vi "Tab Key Process.vi"(4 "CurPage Ctrl #n":refnum<vi>, 5 "Char":i16, 6 "CurPage Ctrl #1":refnum<vi>, 7 "Shift":bool, 9 "Help":refnum<vi>, 10 "Next":refnum<vi>, 11 "Back":refnum<vi>) -> (3 "Discard Key Down Event?":bool)   [LabVIEW 2021]
uses:
  <vilib>/Utility/traverseref.llb/TRef TravTarget.ctl
  <vilib>/Utility/traverseref.llb/VI Scripting - Traverse.lvlib
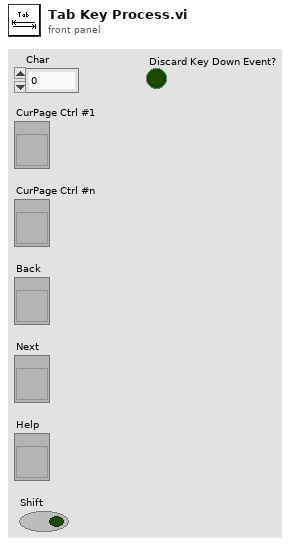
[diagram p1: front panel]
types:
  T1 = typedef "TRef TravTarget.ctl" = enum16{"FP", "BD", "Other"}
  T2 = enum8{"Enabled", "Disabled", "Disabled and Grayed Out"}
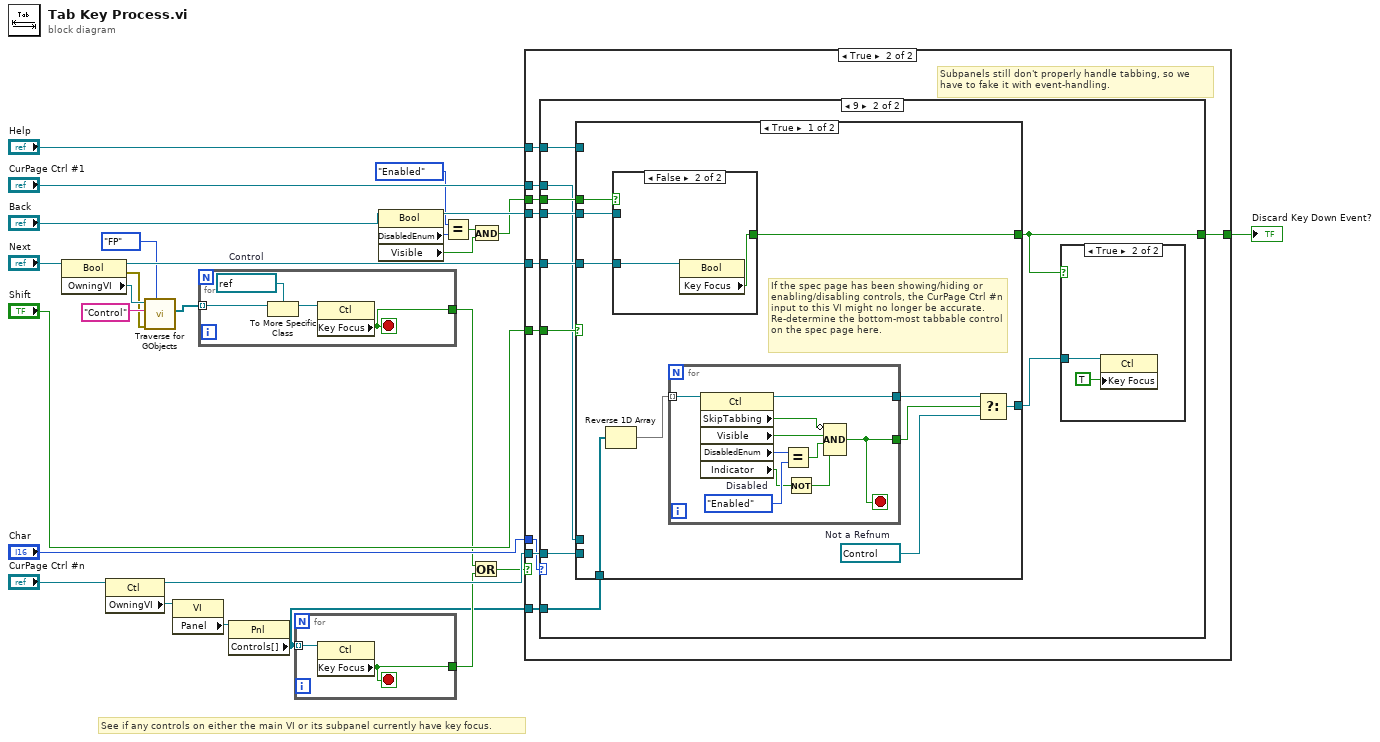
[diagram p0: block diagram]
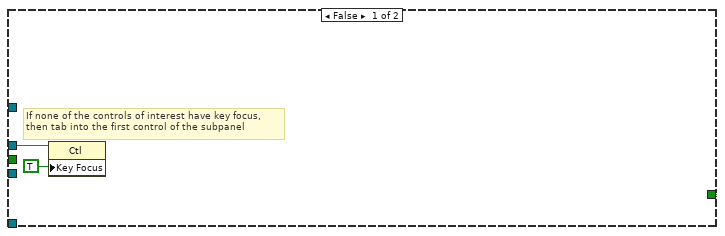
[diagram p2: hidden frame]
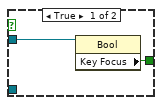
[diagram p5: hidden frame]
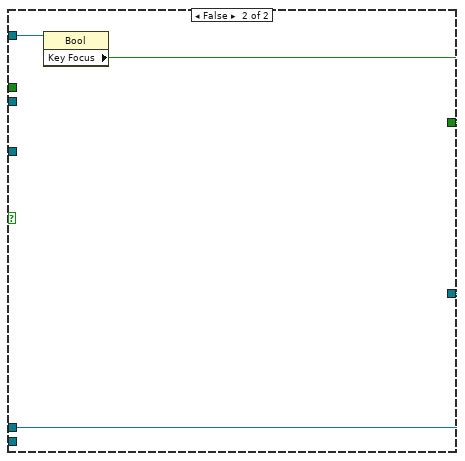
[diagram p6: hidden frame]
diagram:
  # "See if any controls on either the main VI or its subpanel currently have key focus."
  n1 = property class="Bool"(reference="Next") -> (reference out=w13:refnum<vi>, error out=w3:errorcluster, "OwningVI"=w6:refnum<vi>)  [unwired: 1 in]
  n2 = property class="Ctl"(reference="CurPage Ctrl #n") -> (reference out=w12:refnum<vi>, "OwningVI"=w10:refnum<vi>)  [unwired: 1 in, 1 out]
  n3 = call <vilib>:"Traverse for GObjects.vi"("Traverse Target"=TRef_TravTarget."FP", "error in (no error)"=w3, "Class Name"="Control", "VI Refnum"=w6) -> ("References"=w2:refnum<vi>[])  [unwired: 4 in, 3 out]
  n4 = property class="VI"(reference=w10) -> ("Panel"=w11:refnum<vi>)  [unwired: 1 in, 2 out]
  n5 = for {
    tunnel: w2 -> [w29] mode=indexing
    tunnel: [w31] -> w8
    stop <- w31 stop-if-true
    w30 = refnum<vi> refnum  # Control
    n6 = To More Specific Class(target class=w30, reference=w29) -> (specific class reference=w28:refnum<vi>)  [unwired: 1 in, 1 out]
    n7 = property class="Ctl"(reference=w28) -> ("Key Focus"=w31:bool)  [unwired: 1 in, 2 out]
  }
  n8 = property class="Pnl"(reference=w11) -> ("Controls[]"=w1:refnum<vi>[])  [unwired: 1 in, 2 out]
  n9 = for {
    tunnel: w1 -> [w33] mode=indexing
    tunnel: [w32] -> w9
    stop <- w32 stop-if-true
    n10 = property class="Ctl"(reference=w33) -> ("Key Focus"=w32:bool)  [unwired: 1 in, 2 out]
  }
  n11 = property on="Property Node" class="Bool"(reference="Back") -> (reference out=w23:refnum<vi>, "DisabledEnum"=w17:T2, "Visible"=w20:bool)  [unwired: 1 in, 1 out]
  n12 = Equal?(x=T2."Enabled", y=w17) -> (x = y?=w19:bool)
  n13 = Or(x=w8, y=w9) -> (x .or. y?=w7:bool)
  n14 = And(x=w19, y=w20) -> (x .and. y?=w21:bool)
  n15 = case shown="True" w7 {
    tunnel: "CurPage Ctrl #1" -> [w36 w46]
    tunnel: w12 -> [_ w45]
    tunnel: "Help" -> [_ w44]
    tunnel: w13 -> [_ w43]
    tunnel: w23 -> [_ w42]
    tunnel: w21 -> [_ w41]
    tunnel: [TRUE ("Key Focus") w40] -> w16
    tunnel: "Shift" -> [_ w39]
    tunnel: "Char" -> [_ w38]
    tunnel: w1 -> [_ w37]
    frame False {
      # "If none of the controls of interest have key focus,\nthen tab into the first control of the subpanel"
      n16 = property class="Ctl"(reference=w36, "Key Focus"=TRUE) -> ()  [unwired: 1 in, 2 out]
    }
    frame True {
      # "Subpanels still don't properly handle tabbing, so we\nhave to fake it with event-handling."
      n17 = case shown="9" w38 {
        tunnel: w39 -> [_ w56]
        tunnel: [_ w55] -> w40
        tunnel: w41 -> [_ w53]
        tunnel: w42 -> [_ w52]
        tunnel: w43 -> [_ w51]
        tunnel: w44 -> [_ w50]
        tunnel: w45 -> [_ w49]
        tunnel: w46 -> [_ w48]
        tunnel: w37 -> [_ w47]
        frame Default {
        }
        frame 9 {
          n18 = case shown="True" w56 {
            tunnel: [w67 w85] -> w55
            tunnel: [w60 w83] -> w54
            tunnel: w53 -> [w68 _]
            tunnel: w52 -> [w66 _]
            tunnel: w51 -> [w65 _]
            tunnel: w50 -> [_ w84]
            tunnel: w49 -> [_ _]
            tunnel: w48 -> [_ w83]
            tunnel: w47 -> [w64 _]
            frame True {
              w63 = refnum<vi> refnum  # Not a Refnum
              # "If the spec page has been showing/hiding or enabling/disabling controls, the CurPage Ctrl #n input to this VI might no longer be accurate. Re-determine the bottom-most tabbable control on the spec page here."
              n19 = Reverse 1D Array(array=w64) -> (reversed array=w59:refnum<vi>[])
              n20 = case shown="False" w68 {
                tunnel: [w80 w82] -> w67
                tunnel: w66 -> [w79 _]
                tunnel: w65 -> [_ w81]
                frame True {
                  n21 = property on="Property Node" class="Bool"(reference=w79) -> ("Key Focus"=w80:bool)  [unwired: 1 in, 2 out]
                }
                frame False {
                  n22 = property on="Property Node" class="Bool"(reference=w81) -> ("Key Focus"=w82:bool)  [unwired: 1 in, 2 out]
                }
              }
              n23 = for {
                tunnel: [w73] -> w61
                tunnel: [w74] -> w62
                tunnel: w59 -> [w72] mode=indexing
                stop <- w74 stop-if-true
                w77 = T2."Enabled"  # Disabled
                n24 = property class="Ctl"(reference=w72) -> (reference out=w73:refnum<vi>, "SkipTabbing"=w76:bool, "Visible"=w75:bool, "DisabledEnum"=w78:T2, "Indicator"=w70:bool)  [unwired: 1 in, 1 out]
                n25 = Equal?(x=w78, y=w77) -> (x = y?=w71:bool)
                n26 = Not(x=w70) -> (.not. x?=w69:bool)
                n27 = Compound Arithmetic op=AND(invert w76, w75, w71, w69) -> (w74:bool)
              }
              n28 = Select(t=w61, s=w62, f=w63) -> (s? t:f=w60:refnum<vi>)
            }
            frame False {
              n29 = property on="Property Node" class="Bool"(reference=w84) -> ("Key Focus"=w85:bool)  [unwired: 1 in, 2 out]
            }
          }
          n30 = case shown="True" w55 {
            tunnel: w54 -> [_ w57]
            frame False {
            }
            frame True {
              n31 = property on="Property Node" class="Ctl"(reference=w57, "Key Focus"=TRUE) -> ()  [unwired: 1 in, 2 out]
            }
          }
        }
      }
    }
  }
  "Discard Key Down Event?" <- w16
